vi "Get DateTimeOrginal.vi"(8 "error in":errorcluster, 11 "Path":path) -> (0 "error out":errorcluster, 1 "standard error":string, 3 "output 1":timestamp=timestamp(3382438998 s since 1904-01-01))   [LabVIEW 2023, in "EXIF Modifier.lvlib"]
uses:
  EXIF Modifier.lvlib
  <vilib>/Utility/error.llb/Trim Whitespace One-Sided.vi
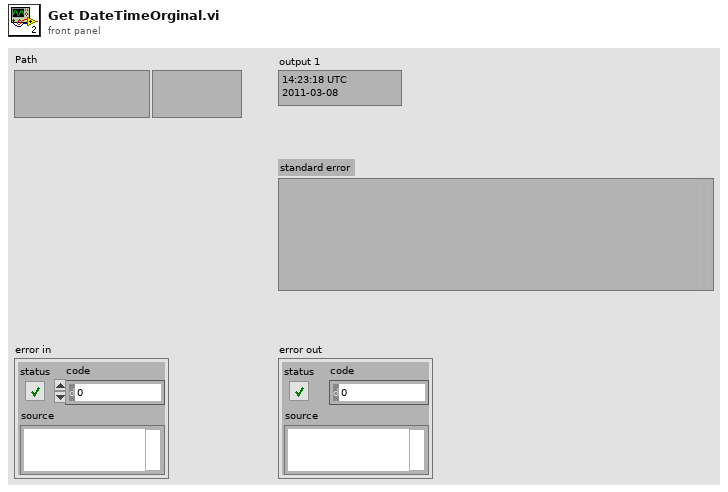
[diagram p1: front panel]
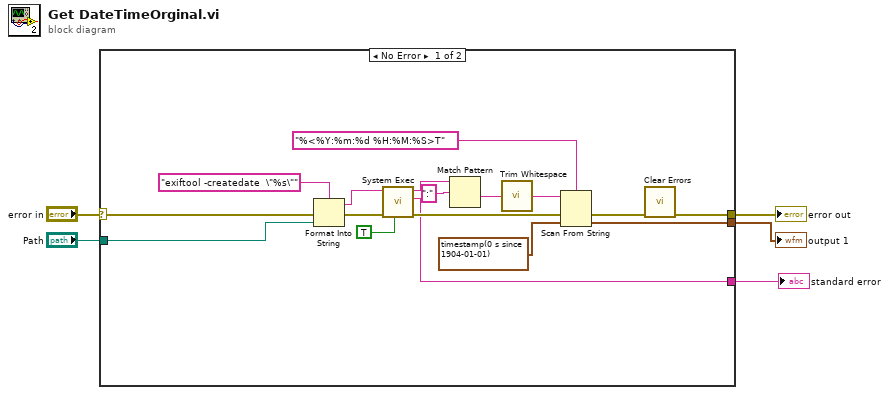
[diagram p0: block diagram]
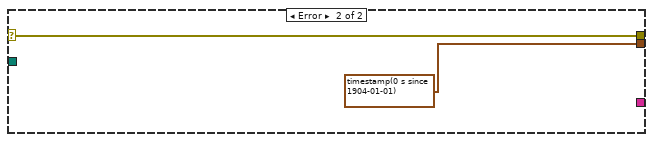
[diagram p2: hidden frame]
diagram:
  n1 = case shown="No Error" "error in" {
    selector: "error in" -> [w9 w24]
    tunnel: [w17 timestamp(0 s since 1904-01-01)] -> w5
    tunnel: "Path" -> [w15 _]
    tunnel: [w6 w24] -> w3
    tunnel: [w8 _] -> w1
    frame No Error {
      n2 = Format Into String(format string="exiftool -createdate  \"%s\"" ("command line"), error in=w9, w15) -> (resulting string=w13:string, error out=w11:errorcluster)  [unwired: 1 in]
      n3 = call <vilib>:"System Exec.vi"("run minimized? (F)"=TRUE, "error in (no error)"=w11, "command line"=w13) -> ("error out"=w10:errorcluster, "standard error"=w8:string, "standard output"=w21:string)  [unwired: 5 in, 1 out]
      n4 = Match Pattern(string=w21, regular expression=":") -> (after substring=w19:string)  [unwired: 1 in, 3 out]
      n5 = call <vilib>:"Trim Whitespace.vi"("string"=w19) -> ("trimmed string"=w16:string)  [unwired: 1 in]
      n6 = Scan From String(format string="%<%Y:%m:%d %H:%M:%S>T", input string=w16, error in=w10, default 1=timestamp(0 s since 1904-01-01)) -> (error out=w12:errorcluster, output 1=w17:timestamp)  [unwired: 1 in, 2 out]
      n7 = call <vilib>:"Clear Errors.vi"("error in (no error)"=w12) -> ("error out"=w6:errorcluster)  [unwired: 5 in, 1 out]
    }
    frame Error {
    }
  }
  "output 1" <- w5
  "error out" <- w3
  "standard error" <- w1
